vi "Read UserDefined State.vi"(8 "error in (no error)":errorcluster, 11 "user-defined-state in":refnum<class "user-defined-state.lvclass">) -> (0 "error out":errorcluster, 2 "state":refnum<class "state.lvclass">, 3 "user-defined-state out":refnum<class "user-defined-state.lvclass">)   [LabVIEW 2020, in "eos.lvlib" / "user-defined-state.lvclass"]
uses:
  user-defined-state.lvclass
  interfaces/state/state.lvclass
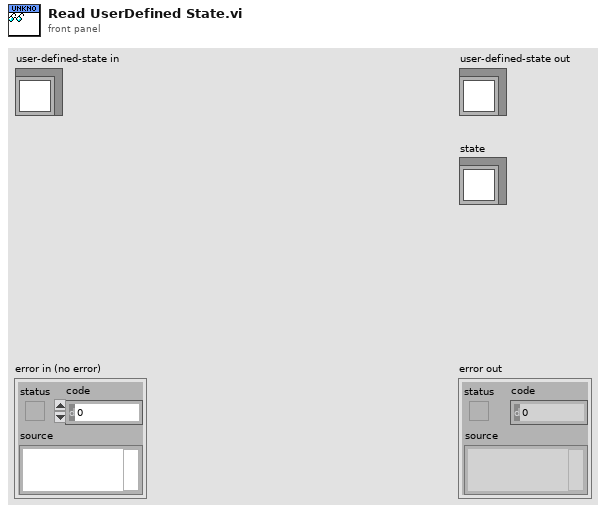
[diagram p1: front panel]
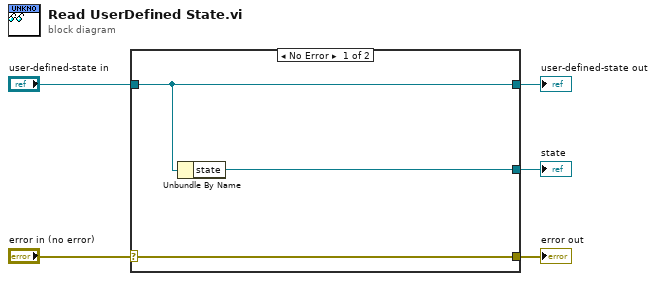
[diagram p0: block diagram]
diagram:
  n1 = case shown="No Error" "error in (no error)" {
    selector: "error in (no error)" -> [w8 w9]
    tunnel: [w8 w9] -> w4
    tunnel: [w7 w10] -> w2
    tunnel: "user-defined-state in" -> [w7 w10]
    tunnel: [w6 _] -> w1
    frame No Error {
      n2 = Unbundle By Name(w7) -> ("state"=w6:refnum<class "state.lvclass">)
    }
    frame Error {
    }
  }
  "error out" <- w4
  "user-defined-state out" <- w2
  "state" <- w1
